vi "HRR-ccw_ang.vi"() -> ()   [LabVIEW 2019]
uses:
  <vilib>/FPGAPlugInAG/myRIO-1900/niLvFpga_Open_myRIO-1900.vi
  <vilib>/rvi/interface/common/dynamic/niFpgaDynamicAddResources.vi
  <vilib>/myRIO/Common/Instrument Driver Framework/Utilities/vis/FPGA Ref Manager.vi
  <vilib>/Utility/error.llb/Error Cluster From Error Code.vi
  <vilib>/myRIO/Common/Instrument Driver Framework/Utilities/vis/Ref Counter.vi
  <vilib>/rvi/interface/common/niFpgaWaitOnOcc.vi
  <vilib>/rvi/interface/nirviOpenFPGA/nirviOpenFPGA.xnode
  FPGA Bitfiles/MyRIOFPGATest_FPGATarget_FPGAMainDefault_pJ5Q7Xj1Ujo.lvbitx
  FPGA Main Default.vi
  <vilib>/rvi/interface/nirviMethod/nirviMethod.xnode
  <vilib>/FPGAPlugInAG/Dynamic/niLvFpga_ConfigureFifo_Dynamic.vi
  <vilib>/rvi/errors/niLvFpgaMergeErrorWithErrorCode.vi
  <vilib>/myRIO/Instrument Drivers/Utilities/Utilities.lvlib
panel:
  out "Actual Depth":u32
  in  "Angulo limite anti-horario":u8[](array[numeric])=[0, 0, 0, 0, 0, 0, 0, 0]
  out "FPGA VI Reference Out":refnum<k20>
  out "error out":errorcluster
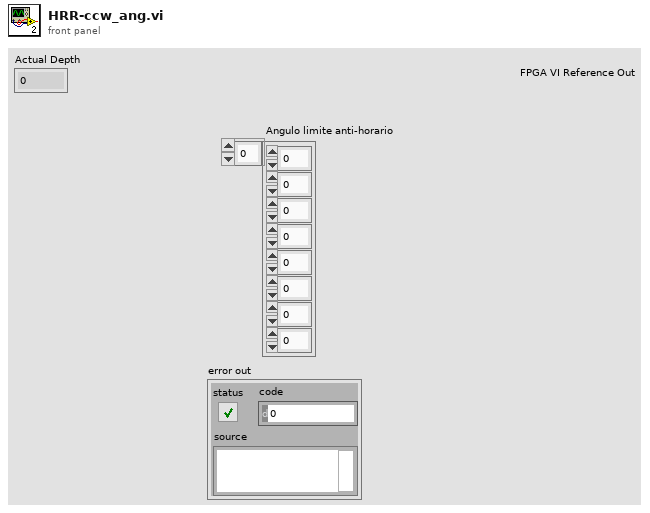
[diagram p1: front panel]
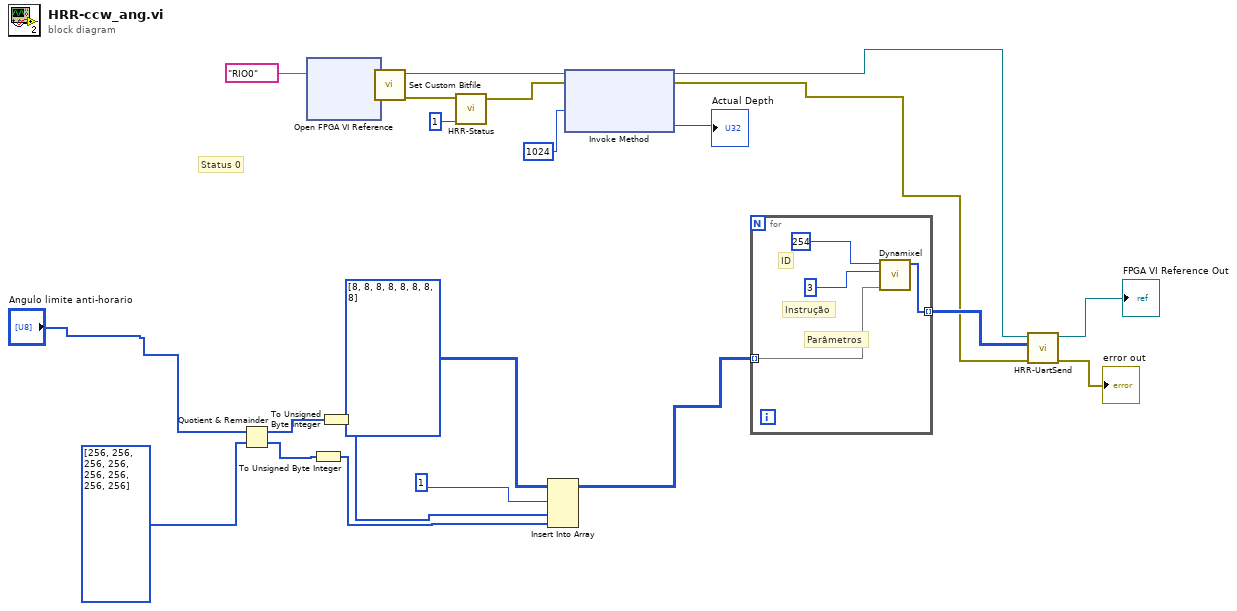
[diagram p0: block diagram]
diagram:
  # "Status 0"
  # "Parâmetros"
  n1 = Quotient & Remainder(x="Angulo limite anti-horario", y=u16[] [256, 256, 256, 256, 256, 256, 256, 256]) -> (x-y*floor(x/y)=w5:u16[], floor(x/y)=w4:u16[])
  n2 = xnode "Open FPGA VI Reference"("resource name"=tag "RIO0") -> ("FPGA VI Reference Out"=w15:refnum<k20>, "error out"=w16:errorcluster)  [unwired: 1 in]
  n3 = To Unsigned Byte Integer(number=w4) -> (unsigned 8bit integer=w2:u8[])
  n4 = To Unsigned Byte Integer(number=w5) -> (unsigned 8bit integer=w3:u8[])
  n5 = call <vilib>:"Set Custom Bitfile.vi"("error in (no error)"=w16, "Custom FPGA Reference In"=w15) -> ("error out"=w9:errorcluster, "Custom FPGA Reference Out"=w10:refnum<k20>)  [unwired: 8 in]
  n6 = call "HRR-Status.vi"("Status (U4)"=u8 1 ("number"), "error in (no error)"=w9) -> ("error out"=w12:errorcluster)  [unwired: 9 in]
  n7 = Insert Into Array(array=u8[][] [[8], [8], [8], [8], [8], [8], [8], [8]], index (col)=1 ("disabled index (col)"), new element #1=w3, new element #2=w2) -> (w21:u8[][])  [unwired: 1 in]
  n8 = xnode "Invoke Method"("FPGA VI Reference In"=w10, "error in"=w12, "Requested Depth"=u32 1024) -> ("FPGA VI Reference Out"=w7:refnum<k20>, "error out"=w8:errorcluster, "Actual Depth"=→"Actual Depth":u32)
  n9 = for {
    tunnel: w21 -> [w25] mode=indexing
    tunnel: [w24] -> w18 mode=indexing
    # "Instrução"
    # "ID"
    n10 = call "Dynamixel.vi"("ID"=u8 254, "Instruction"=u8 3, "Array in"=w25) -> ("Array out"=w24:u8[])  [unwired: 7 in]
  }
  n11 = call "HRR-UartSend.vi"("error in (no error)"=w8, "Array"=w18, "Refnum in"=w7) -> ("error out"=→"error out":errorcluster, "Refnum out"=→"FPGA VI Reference Out":refnum<k20>)  [unwired: 7 in]
